vi "Generate Multiplication Table.vi"(8 "Stop Application":bool, 9 "Clear Tables":bool, 10 "Get Tables":bool, 11 "Table Number":i32) -> (3 "Respective Multiplication Table":string[][](table))   [LabVIEW 2020]
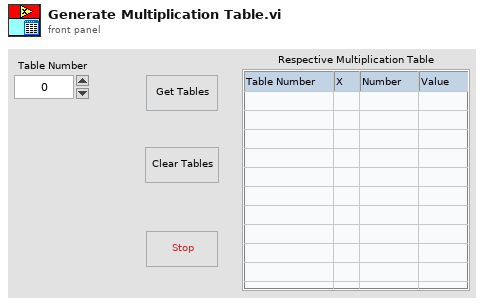
[diagram p1: front panel]
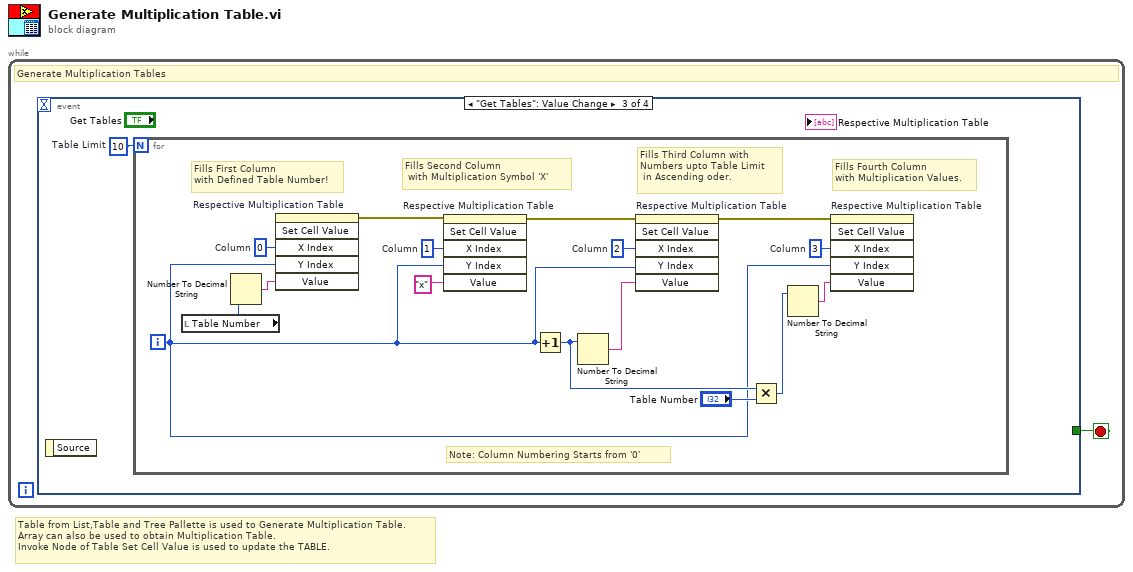
[diagram p0: block diagram]
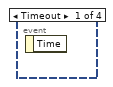
[diagram p2: hidden frame]
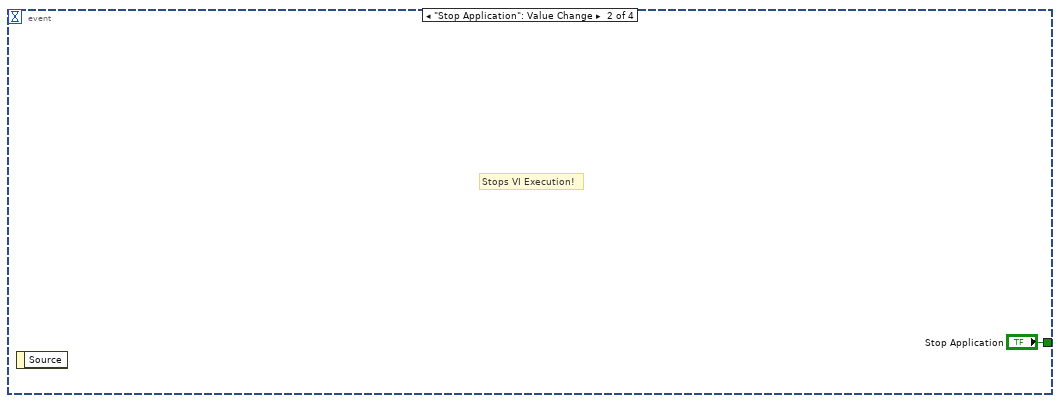
[diagram p3: hidden frame]
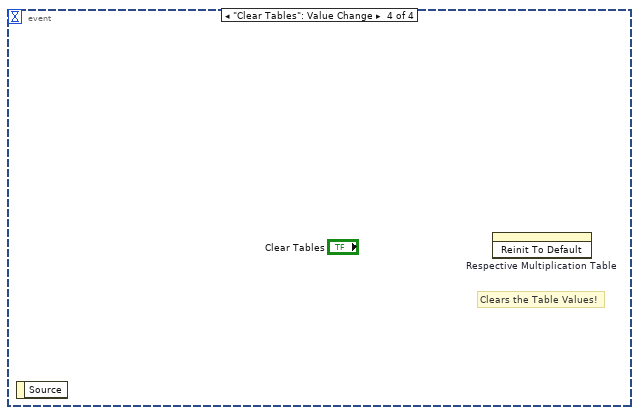
[diagram p4: hidden frame]
diagram:
  # "Table from List,Table and Tree Pallette is used to Generate Multiplication Table. \nArray can also be used to obtain Multiplication Table.\nInvoke Node of Table Set Cell Value is used to update the TABLE."
  n1 = while {
    stop <- w1 stop-if-true
    # "Generate Multiplication Tables"
    n2 = event shown="[2] \"Get Tables\": Value Change" {
      selector: _ -> [_ _ _ _]
      dyn-events: _ -> [_ _ _ _]
      timeout: _ -> [_ _ _ _]
      tunnel: [_ "Stop Application" _ _] -> w1
      event Timeout {
        n3 = event-data() -> ()  [unwired: 1 in, 1 out]
      }
      event "Stop Application": Value Change {
        # "Stops VI Execution!"
        n4 = event-data() -> ()  [unwired: 1 in, 1 out]
      }
      event "Get Tables": Value Change {
        w3 = 10  # Table Limit
        n5 = event-data() -> ()  [unwired: 1 in, 1 out]
        n6 = for {
          N: w3 -> [_]
          i -> [w7]
          w14 = 3  # Column
          w16 = 2  # Column
          w18 = 1  # Column
          w19 = 0  # Column
          # "Note: Column Numbering Starts from '0'"
          # "Fills Fourth Column \nwith Multiplication Values."
          # "Fills Third Column with \nNumbers upto Table Limit\n in Ascending oder."
          # "Fills Second Column\n with Multiplication Symbol 'X'"
          # "Fills First Column  \nwith Defined Table Number!"
          n7 = local read "Table Number"() -> (w10:i32)
          n8 = Number To Decimal String(number=w10) -> (decimal integer string=w9:string)  [unwired: 1 in]
          n9 = invoke on="Respective Multiplication Table" class="Tbl (strict)" method="Set Cell Value"("X Index"=w19, "Y Index"=w7, "Value"=w9) -> (error out=w6:errorcluster)  [unwired: 3 in, 5 out]
          n10 = invoke on="Respective Multiplication Table" class="Tbl (strict)" method="Set Cell Value"(error in=w6, "X Index"=w18, "Y Index"=w7, "Value"="x") -> (error out=w5:errorcluster)  [unwired: 2 in, 5 out]
          n11 = Increment(x=w7) -> (x+1=w8:i32)
          n12 = Number To Decimal String(number=w8) -> (decimal integer string=w15:string)  [unwired: 1 in]
          n13 = invoke on="Respective Multiplication Table" class="Tbl (strict)" method="Set Cell Value"(error in=w5, "X Index"=w16, "Y Index"=w7, "Value"=w15) -> (error out=w4:errorcluster)  [unwired: 2 in, 5 out]
          n14 = Multiply(x=w8, y="Table Number") -> (x*y=w12:i32)
          n15 = Number To Decimal String(number=w12) -> (decimal integer string=w11:string)  [unwired: 1 in]
          n16 = invoke on="Respective Multiplication Table" class="Tbl (strict)" method="Set Cell Value"(error in=w4, "X Index"=w14, "Y Index"=w7, "Value"=w11) -> ()  [unwired: 2 in, 6 out]
        }
      }
      event "Clear Tables": Value Change {
        # "Clears the Table Values!"
        n17 = event-data() -> ()  [unwired: 1 in, 1 out]
        n18 = invoke on="Respective Multiplication Table" class="Tbl (strict)" method="Reinit To Default"() -> ()  [unwired: 3 in, 3 out]
      }
    }
  }
